vi "subDFD_Set Control Value by Name.vi"(8 "error in (no error)":errorcluster, 9 "Value":variant, 10 "control name":string, 11 "vi reference in":refnum<vi>) -> (0 "error out":errorcluster, 3 "vi reference out":refnum<vi>)   [LabVIEW 2017]
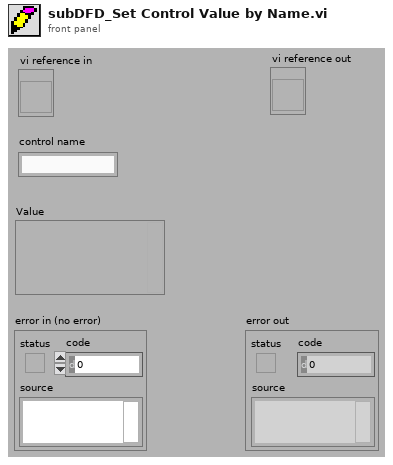
[diagram p1: front panel]
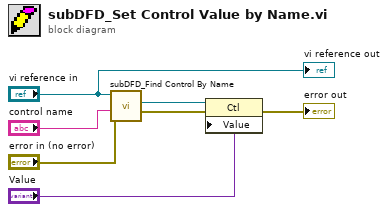
[diagram p0: block diagram]
diagram:
  n1 = call <vilib>:"subDFD_Find Control By Name.vi"("error in (no error)"="error in (no error)", "control name"="control name", "vi refnum in"="vi reference in") -> ("error out"=w2:errorcluster, "control refnum"=w3:refnum<vi>)  [unwired: 1 in, 6 out]
  n2 = property class="Ctl"(reference=w3, error in=w2, "Value"="Value") -> (error out=→"error out":errorcluster)  [unwired: 1 out]
  "vi reference out" <- "vi reference in"
